vi "TCP Loop - Server as Producer.vi"(6 "params":T2={"Open timeout(ms)"=50, "Trans timeout(ms)"=200, "idle time(ms)"=100}, 7 "Discard Data when not connected?(T)":bool=TRUE, 8 "Error In":errorcluster, 9 "port":u16=4008, 10 "Server Name":string, 11 "DataQueue":refnum<queue>) -> (0 "Error Out":errorcluster)   [LabVIEW 2017]
doc: "TCP transmission loop acting as the server. It listens on port and sends the strings taken from DataQueue to the connected client. Set Discard Data when not connected?(T) to drop data while no client is attached."
panel:
  out "idle time(ms)":u32
  out "remote port":u16
  out "remote address":string
  out "STATE":T1(ring)
  out "current time":timestamp
  out "data value":T3={"stopped?"=FALSE, "started?"=FALSE, "re-inited?"=FALSE, "Connected?"=FALSE, "transmit?"=FALSE, "bytes written"=0, "#in queue"=0, "Open timeout(ms)"=50, "Trans timeout(ms)"=1000, "idle time(ms)"=1000}
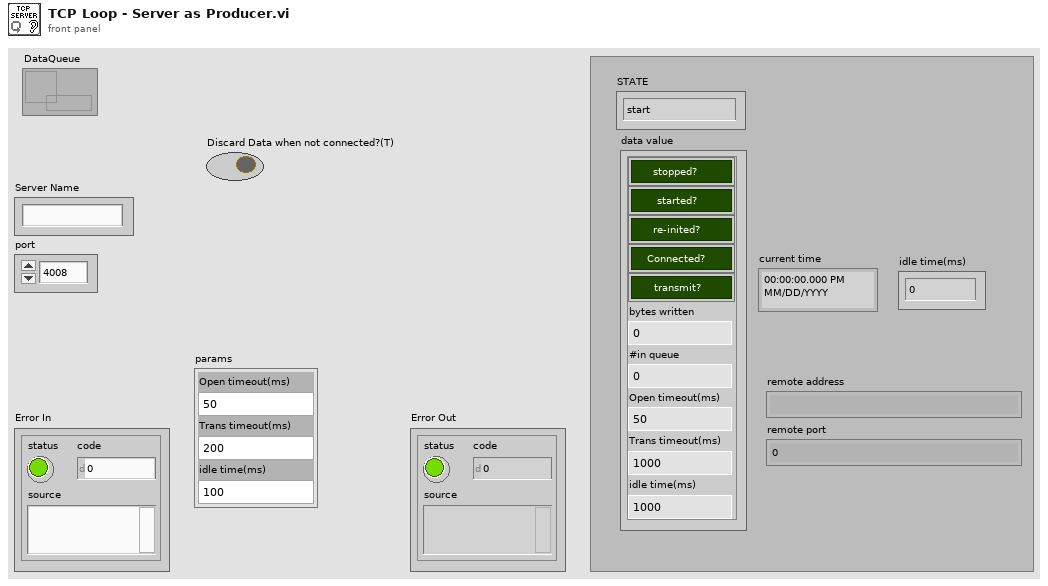
[diagram p1: front panel]
types:
  T1 = enum16{"start", "connect", "work", "close", "stop loop"}
  T2 = cluster{"Open timeout(ms)":i32, "Trans timeout(ms)":i32, "idle time(ms)":i32}
  T3 = cluster{"stopped?":bool, "started?":bool, "re-inited?":bool, "Connected?":bool, "transmit?":bool, "bytes written":i32, "#in queue":i32, "Open timeout(ms)":i32, "Trans timeout(ms)":i32, "idle time(ms)":i32}
  T4 = cluster{"data value reference":refnum<data-value>, "data ref err":errorcluster}
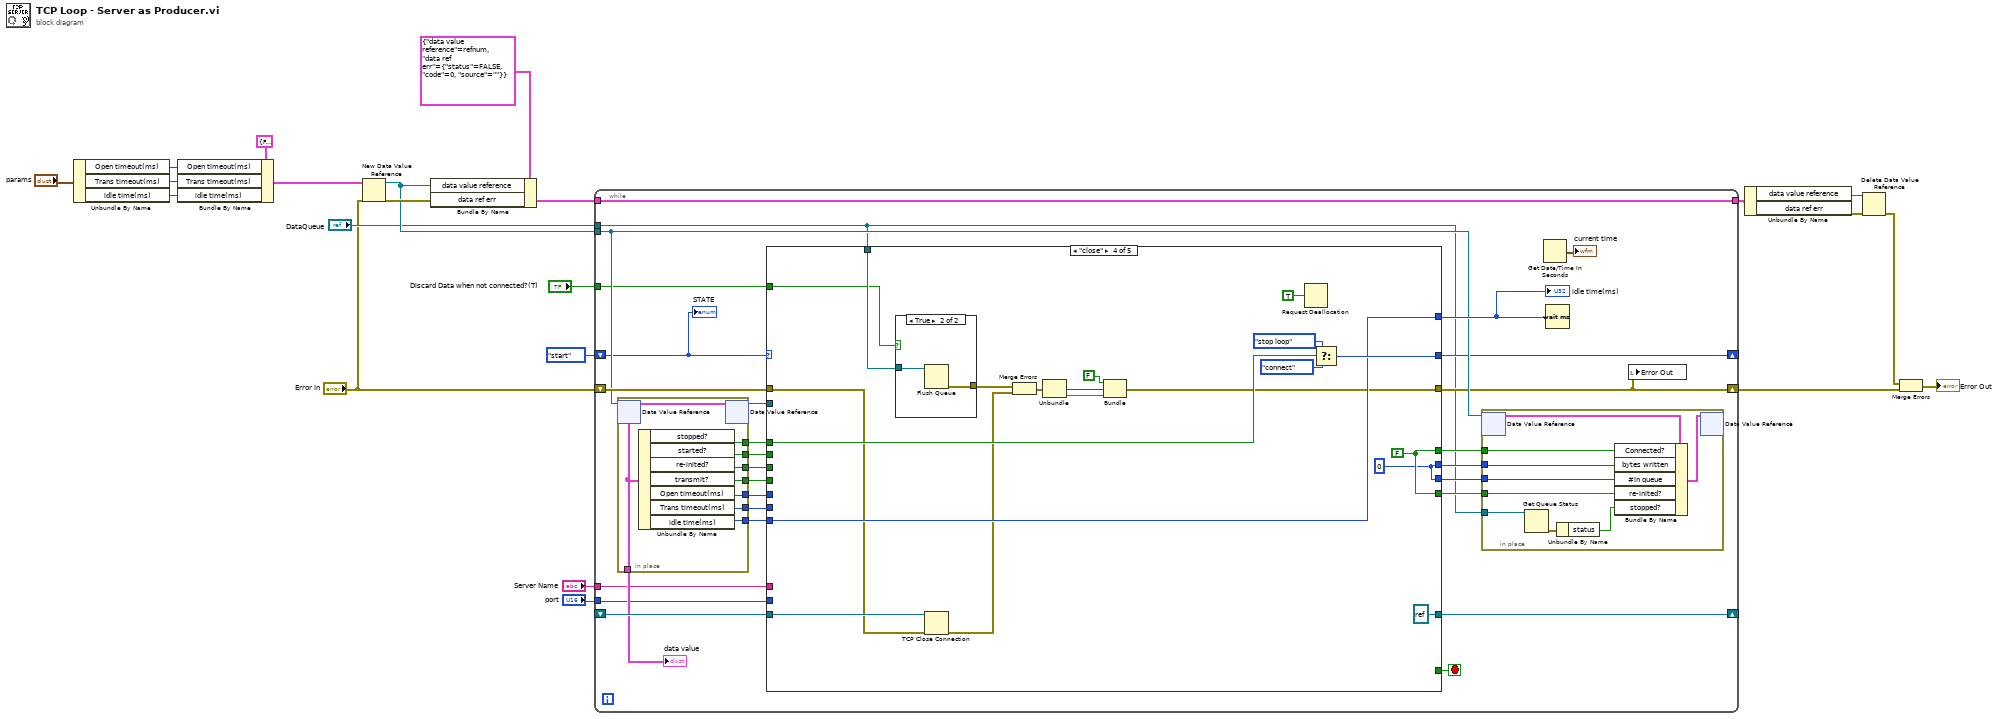
[diagram p0: block diagram]
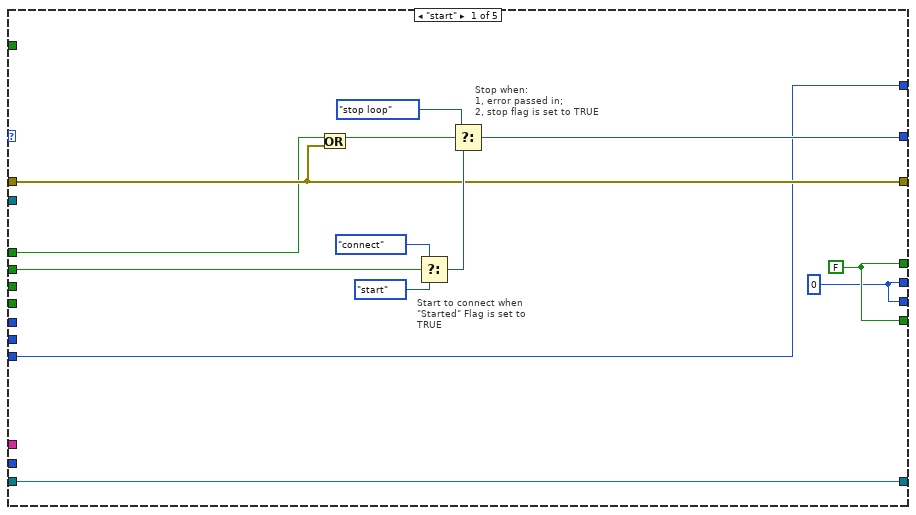
[diagram p2: hidden frame]
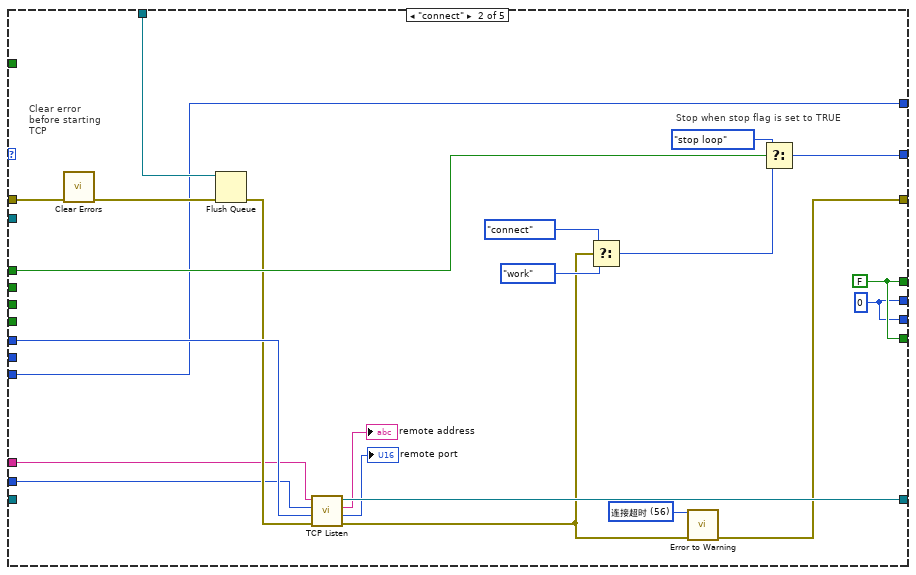
[diagram p3: hidden frame]
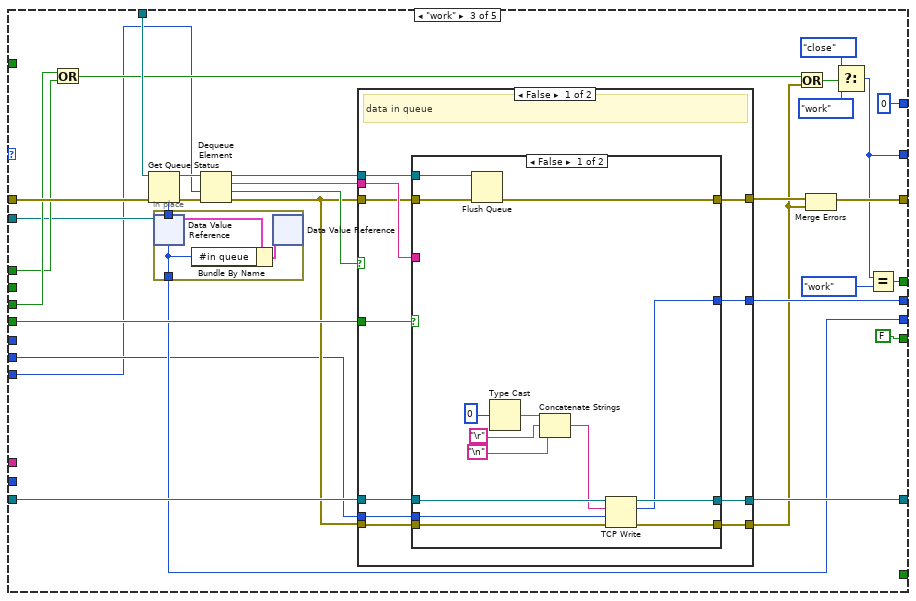
[diagram p4: hidden frame]
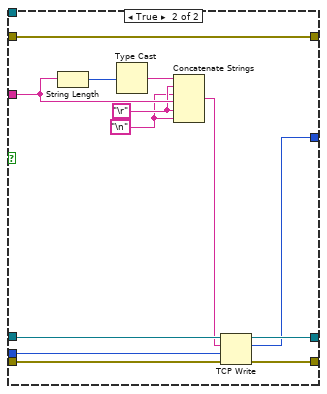
[diagram p5: hidden frame]
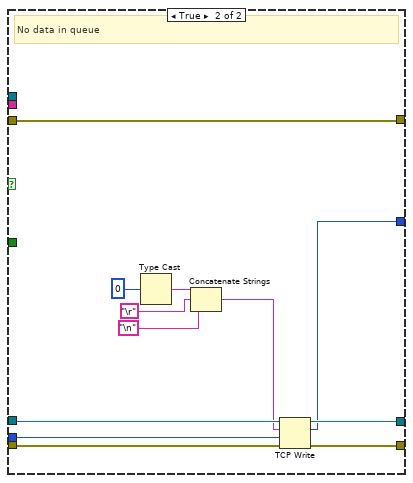
[diagram p6: hidden frame]
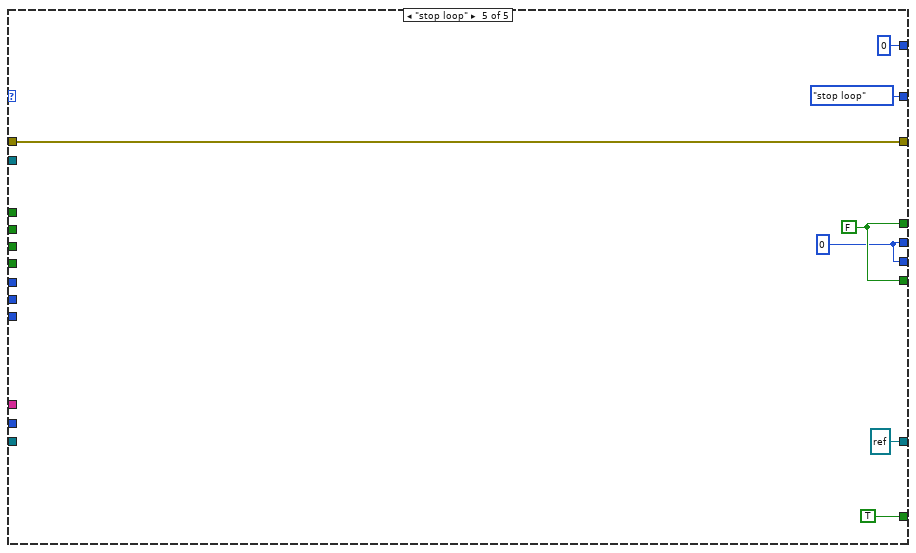
[diagram p8: hidden frame]
diagram:
  n1 = Unbundle By Name("params") -> ("Open timeout(ms)"=w9:i32, "Trans timeout(ms)"=w8:i32, "idle time(ms)"=w7:i32)
  n2 = Bundle By Name(cluster=T3 {"stopped?"=FALSE, "started?"=TRUE, "re-inited?"=FALSE, "Connected?"=FALSE, "transmit?"=TRUE, "bytes written"=0, "#in queue"=0, "Open timeout(ms)"=50, "Trans timeout(ms)"=0, "idle time(ms)"=0} ("TCP Params"), "Open timeout(ms)"=w9, "Trans timeout(ms)"=w8, "idle time(ms)"=w7) -> (w6:T3)
  n3 = New Data Value Reference(data value=w6, error in="Error In") -> (data value reference=w17:refnum<data-value>, error out=w20:errorcluster)
  n4 = Bundle By Name(cluster=T4 {"data value reference"=refnum, "data ref err"={"status"=FALSE, "code"=0, "source"=""}}, "data value reference"=w17, "data ref err"=w20) -> (w19:T4)
  n5 = while {
    shift-right: [w32] -> _
    shift-left: T1."start" -> [w29]
    tunnel: w17 -> [w41]
    shift-right: [w43] -> _
    shift-left: _ -> [w42]
    tunnel: "DataQueue" -> [w26]
    tunnel: w19 -> [w33]
    tunnel: [w33] -> w18
    shift-right: [w27] -> w4
    shift-left: "Error In" -> [w45]
    tunnel: "Server Name" -> [w25]
    tunnel: "port" -> [w24]
    tunnel: "Discard Data when not connected?(T)" -> [w23]
    stop <- w37 stop-if-true
    n6 = in-place {
      in-place-border: [w67] -> w49
      in-place-border: [w66] -> w48
      in-place-border: [w65] -> w47
      in-place-border: [w64] -> w46
      in-place-border: [w63] -> w44
      in-place-border: [w62] -> w36
      in-place-border: [w61] -> w31
      in-place-border: [w60] -> w30
      n7 = in-place-dvr #1(w41) -> (w62:T3)  [unwired: 1 out]
      n8 = Unbundle By Name(w62) -> ("stopped?"=w64:bool, "started?"=w65:bool, "re-inited?"=w66:bool, "transmit?"=w67:bool, "Open timeout(ms)"=w63:i32, "Trans timeout(ms)"=w61:i32, "idle time(ms)"=w60:i32)
      n9 = in-place-dvr #1(w62) -> (w35:refnum<data-value>)  [unwired: 1 out]
    }
    "data value" <- w36
    n10 = case shown="\"close\"" w29 {
      tunnel: [w71 w86 u32 0 ("idle time(ms)") w197 u32 0] -> w50
      tunnel: w49 -> [_ _ w127 _ _]
      tunnel: w48 -> [_ _ w120 _ _]
      tunnel: w47 -> [w79 _ _ _ _]
      tunnel: w46 -> [w72 w100 w119 w203 _]
      tunnel: w45 -> [w73 w96 w130 w195 w214]
      tunnel: [w80 w99 w115 w204 T1."stop loop"] -> w32
      tunnel: [w73 w83 w121 w191 w214] -> w27
      tunnel: w44 -> [_ w102 _ _ _]
      tunnel: [w77 w101 w123 refnum<k5> refnum ("connection ID") refnum<k5> refnum ("connection ID")] -> w43
      tunnel: w26 -> [_ w95 w131 w206 _]
      tunnel: w42 -> [w77 _ w125 w205 _]
      tunnel: [w76 w97 w116 w202 w213] -> w40
      tunnel: [w76 w97 FALSE w202 w213] -> w39
      tunnel: [w75 w93 w114 w200 w211] -> w38
      tunnel: [_ _ _ _ TRUE] -> w37
      tunnel: w35 -> [_ _ w110 _ _]
      tunnel: [w75 w93 w109 w200 w211] -> w34
      tunnel: w31 -> [_ _ w108 _ _]
      tunnel: w30 -> [w71 w86 w104 w197 _]
      tunnel: w25 -> [_ w81 _ _ _]
      tunnel: w24 -> [_ w82 _ _ _]
      tunnel: w23 -> [_ _ _ w187 _]
      frame "start" {
        w75 = 0 ("bytes written")
        w76 = FALSE
        # "Stop when:\n1, error passed in;\n2, stop flag is set to TRUE"
        # "Start to connect when \"Started\" Flag is set to TRUE"
        n11 = Or(x=w72, y=w73) -> (x .or. y?=w74:bool)
        n12 = Select(t=T1."connect", s=w79, f=T1."start") -> (s? t:f=w78:T1)
        n13 = Select(t=T1."stop loop", s=w74, f=w78) -> (s? t:f=w80:T1)
      }
      frame "connect" {
        w85 = 56 items=["无错误", "参数错误", "内存已满", "超出区域", "文件结束", "文件已打开", "一般文件IO错误", "未找到文件", "文件权限错误", "磁盘已满", "路径副本", "打开过多文件", "未启用", "未找到资源文件", "无法添加资源", "未找到资源", "未找到图像", "图像内存错误", "画笔不存在", "配置错误类型", "配置未找到解析段", "配置解析错误", "配置内存错误", "错误外部代码格式", "错误外部代码偏移量", "外部代码不存在", "空窗口", "销毁窗口错误", "空菜单", "打印已中止", "错误打印记录", "打印驱动程序错误", "打印时窗口错误", "打印时内存错误", "打印对话框错误", "一般打印错误", "无效设备引用句柄", "设备未找到", "设备参数错误", "设备单位错误", "无法打开设备", "设备调用已中止", "一般错误", "用户已取消", "对象ID过低", "对象ID过高", "对象不在堆中", "未知的堆", "错误DefProc ID", "DefProc不在表格中", "范围外信息", "空方法", "未知信息", "不支持管理器调用", "错误地址", "连接过程中", "连接超时", "连接过程中", "不支持网络属性", "网络错误", "正在使用的地址", "系统缺少内存", "连接已中止", "连接已拒绝", "连接未建立", "连接已建立", "连接已关闭", "初始化错误（交互应用程序管理器）", "错误事件发生", "等待无约束事件发生处理程序", "事件发生队列溢出", "错误路径", "未发出信号量", "未识别类型（交互应用程序管理器）"] ("2nd Error to Convert")
        w93 = 0
        w97 = FALSE
        # "Clear error before starting TCP"
        # "Stop when stop flag is set to TRUE"
        n14 = call <vilib>:"Clear Errors.vi"("error in (no error)"=w96) -> ("error out"=w89:errorcluster)  [unwired: 5 in, 1 out]
        n15 = Flush Queue(queue=w95, error in (no error)=w89) -> (error out=w94:errorcluster)  [unwired: 2 out]
        n16 = call <vilib>:"TCP Listen.vi"("error in (no error)"=w94, "timeout ms (wait forever: -1)"=w102, "port"=w82, "service name"=w81) -> ("error out"=w84:errorcluster, "remote port"=→"remote port":u16, "remote address"=→"remote address":string, "connection ID"=w101:refnum<k5>)  [unwired: 3 in, 1 out]
        n17 = Select(t=T1."connect", s=w84, f=T1."work") -> (s? t:f=w98:T1)
        n18 = call <vilib>:"Error to Warning.vi"("1st Error to Convert"=w85, "error in"=w84) -> ("warning out"=w83:errorcluster)  [unwired: 13 in]
        n19 = Select(t=T1."stop loop", s=w100, f=w98) -> (s? t:f=w99:T1)
      }
      frame "work" {
        n20 = Or(x=w120, y=w119) -> (x .or. y?=w118:bool)
        n21 = Get Queue Status(queue=w131, error in (no error)=w130) -> (queue out=w132:refnum<queue>, error out=w133:errorcluster, # elements in queue=w111:i32)  [unwired: 1 in, 5 out]
        n22 = in-place {
          in-place-border: w111 -> [w134]
          in-place-border: [w134] -> w109
          n23 = in-place-dvr #2(w110) -> (w136:T3)  [unwired: 1 out]
          n24 = Bundle By Name(cluster=w136, "#in queue"=w134) -> (w135:T3)
          n25 = in-place-dvr #2(w135) -> ()  [unwired: 2 out]
        }
        n26 = Dequeue Element(queue=w132, timeout in ms (-1)=w104, error in (no error)=w133) -> (queue out=w129:refnum<queue>, element=w128:string, timed out?=w126:bool, error out=w124:errorcluster)
        n27 = case shown="False" w126 {
          tunnel: w125 -> [w146 w179]
          tunnel: w124 -> [w145 w181]
          tunnel: [w147 w178] -> w123
          tunnel: [w144 w180] -> w112
          tunnel: [w139 w186] -> w122
          tunnel: [w143 w176] -> w114
          tunnel: w124 -> [w140 w186]
          tunnel: w129 -> [w141 _]
          tunnel: w128 -> [w142 _]
          tunnel: w127 -> [w138 _]
          tunnel: w108 -> [w137 w175]
          frame False {
            # "data in queue"
            n28 = case shown="False" w138 {
              tunnel: [w158 w174] -> w147
              tunnel: [w157 w173] -> w144
              tunnel: w146 -> [w159 w172]
              tunnel: w145 -> [w160 w171]
              tunnel: w142 -> [_ w168]
              tunnel: [w156 w170] -> w143
              tunnel: w137 -> [w155 w166]
              tunnel: w141 -> [w154 _]
              tunnel: w140 -> [w153 w165]
              tunnel: [w152 w165] -> w139
              frame False {
                n29 = Flush Queue(queue=w154, error in (no error)=w153) -> (error out=w152:errorcluster)  [unwired: 2 out]
                n30 = Type Cast(x=0 ("length")) -> (*(type *) &x=w149:string)  [unwired: 1 in]
                n31 = Concatenate Strings(w149, "\r", "\n") -> (w148:string)
                n32 = TCP Write(connection ID=w159, data in=w148, error in (no error)=w160, 9:w155) -> (connection ID out=w158:refnum<k5>, bytes written=w156:i32, error out=w157:errorcluster)
              }
              frame True {
                w163 = "\r"
                w162 = "\n"
                n33 = String Length(string=w168) -> (length=w169:i32)
                n34 = Type Cast(x=w169) -> (*(type *) &x=w164:string)  [unwired: 1 in]
                n35 = Concatenate Strings(w164, w163, w162, w168, w163, w162) -> (w167:string)
                n36 = TCP Write(connection ID=w172, data in=w167, error in (no error)=w171, 9:w166) -> (connection ID out=w174:refnum<k5>, bytes written=w170:i32, error out=w173:errorcluster)
              }
            }
          }
          frame True {
            # "No data in queue"
            n37 = Type Cast(x=0 ("length")) -> (*(type *) &x=w182:string)  [unwired: 1 in]
            n38 = Concatenate Strings(w182, "\r", "\n") -> (w177:string)
            n39 = TCP Write(connection ID=w179, data in=w177, error in (no error)=w181, 9:w175) -> (connection ID out=w178:refnum<k5>, bytes written=w176:i32, error out=w180:errorcluster)
          }
        }
        n40 = Or(x=w118, y=w112) -> (x .or. y?=w117:bool)
        n41 = Merge Errors(w122, w112) -> (w121:errorcluster)
        n42 = Select(t=T1."close", s=w117, f=T1."work") -> (s? t:f=w115:T1)
        n43 = Equal?(x=w115, y=T1."work") -> (x = y?=w116:bool)
      }
      frame "close" {
        w200 = 0
        w202 = FALSE
        n44 = case shown="True" w187 {
          tunnel: w206 -> [_ w208]
          tunnel: [_ w207] -> w188
          frame False {
          }
          frame True {
            n45 = Flush Queue(queue=w208) -> (error out=w207:errorcluster)  [unwired: 1 in, 2 out]
          }
        }
        n46 = TCP Close Connection(connection ID=w205, error in (no error)=w195) -> (error out=w194:errorcluster)  [unwired: 1 in, 1 out]
        n47 = Merge Errors(w188, w194) -> (w189:errorcluster)
        n48 = Unbundle(w189) -> ("code"=w193:i32, "source"=w192:string)  [unwired: 1 out]
        n49 = Bundle("status"=FALSE, "code"=w193, "source"=w192) -> (w191:errorcluster)  [unwired: 1 in]
        n50 = Request Deallocation(TRUE ("flag")) -> ()
        n51 = Select(t=T1."stop loop", s=w203, f=T1."connect") -> (s? t:f=w204:T1)
      }
      frame "stop loop" {
        w211 = 0 ("bytes written")
        w213 = FALSE
      }
    }
    "idle time(ms)" <- w50
    n52 = in-place {
      in-place-border: w40 -> [w57]
      in-place-border: w39 -> [w55]
      in-place-border: w38 -> [w56]
      in-place-border: w34 -> [w54]
      in-place-border: w26 -> [w51]
      n53 = in-place-dvr #3(w41) -> (w59:T3)  [unwired: 1 out]
      n54 = Get Queue Status(queue=w51) -> (error out=w53:errorcluster)  [unwired: 2 in, 7 out]
      n55 = Unbundle By Name(w53) -> ("status"=w52:bool)
      n56 = Bundle By Name(cluster=w59, "Connected?"=w57, "bytes written"=w56, "#in queue"=w54, "re-inited?"=w55, "stopped?"=w52) -> (w58:T3)
      n57 = in-place-dvr #3(w58) -> ()  [unwired: 2 out]
    }
    n58 = Get Date/Time In Seconds() -> (seconds since 1Jan1904=→"current time":timestamp)
    n59 = Wait (ms)(milliseconds to wait=w50) -> ()  [unwired: 1 out]
    n60 = local write "Error Out"(w27) -> ()
    "STATE" <- w29
  }
  n61 = Unbundle By Name(w18) -> ("data value reference"=w16:refnum<data-value>, "data ref err"=w14:errorcluster)
  n62 = Delete Data Value Reference(data value reference=w16, error in=w14) -> (error out=w13:errorcluster)  [unwired: 1 out]
  n63 = Merge Errors(w13, w4) -> (→"Error Out":errorcluster)
